vi "클러스터.vi"() -> ()   [LabVIEW 2020]
panel:
  out "output cluster":T1
  out "Array 3":bool[](array[boolean])
  out "String 2":string
  out "Boolean 2":bool
  out "Numeric 2":dbl
  out "String 3":string
  out "Numeric 3":dbl
  in  "String":string
  in  "Boolean":bool
  in  "Numeric":dbl
  in  "Array 2":bool[](array[boolean])
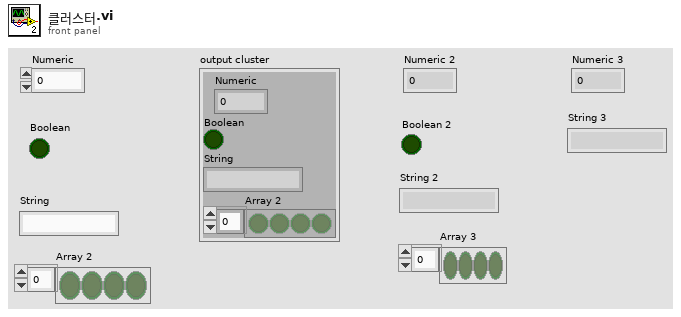
[diagram p1: front panel]
types:
  T1 = cluster{"Numeric":dbl, "Boolean":bool, "String":string, "Array 2":bool[]}
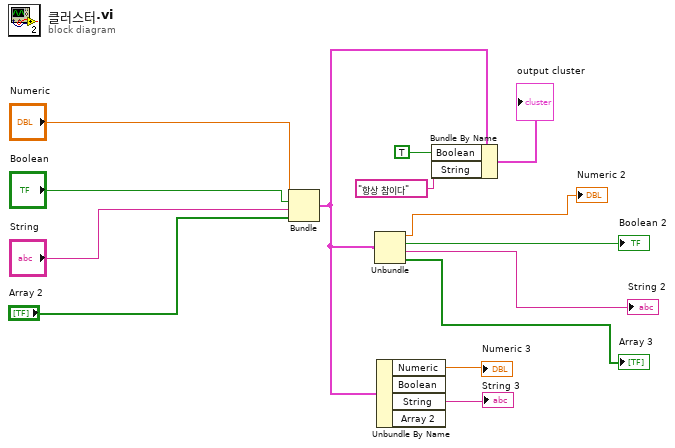
[diagram p0: block diagram]
diagram:
  n1 = Bundle("Numeric"="Numeric", "Boolean"="Boolean", "String"="String", "Array 2"="Array 2") -> (w8:T1)  [unwired: 1 in]
  n2 = Unbundle "Unbundle"(w8) -> ("Numeric"=→"Numeric 2":dbl, "Boolean"=→"Boolean 2":bool, "String"=→"String 2":string, "Array 2"=→"Array 3":bool[])
  n3 = Unbundle By Name "Unbundle By Name"(w8) -> ("Numeric"=→"Numeric 3":dbl, "String"=→"String 3":string)  [unwired: 2 out]
  n4 = Bundle By Name(cluster=w8, "Boolean"=TRUE, "String"="항상 참이다") -> (→"output cluster":T1)
